vi "RTS Build Filename List.vi"(8 "Error In":errorcluster, 11 "RTS Config Setup":T1) -> (0 "Error Out":errorcluster, 3 "Full Filename List":string)   [LabVIEW 2016]
uses:
  Type Definitions/RTS Configuration Setup.ctl
  Type Definitions/RTS Wago Config.ctl
  Type Definitions/RTS APLUS Config.ctl
  Type Definitions/RTS Yokogawa MX Config.ctl
  Type Definitions/RTS Replay Server Control.ctl
  Type Definitions/RTS Server Configuration.ctl
  Type Definitions/RTS Station Settions TCP Comms.ctl
  Type Definitions/RTS Chamber Save Status.ctl
  Type Definitions/RTS Test Pattern.ctl
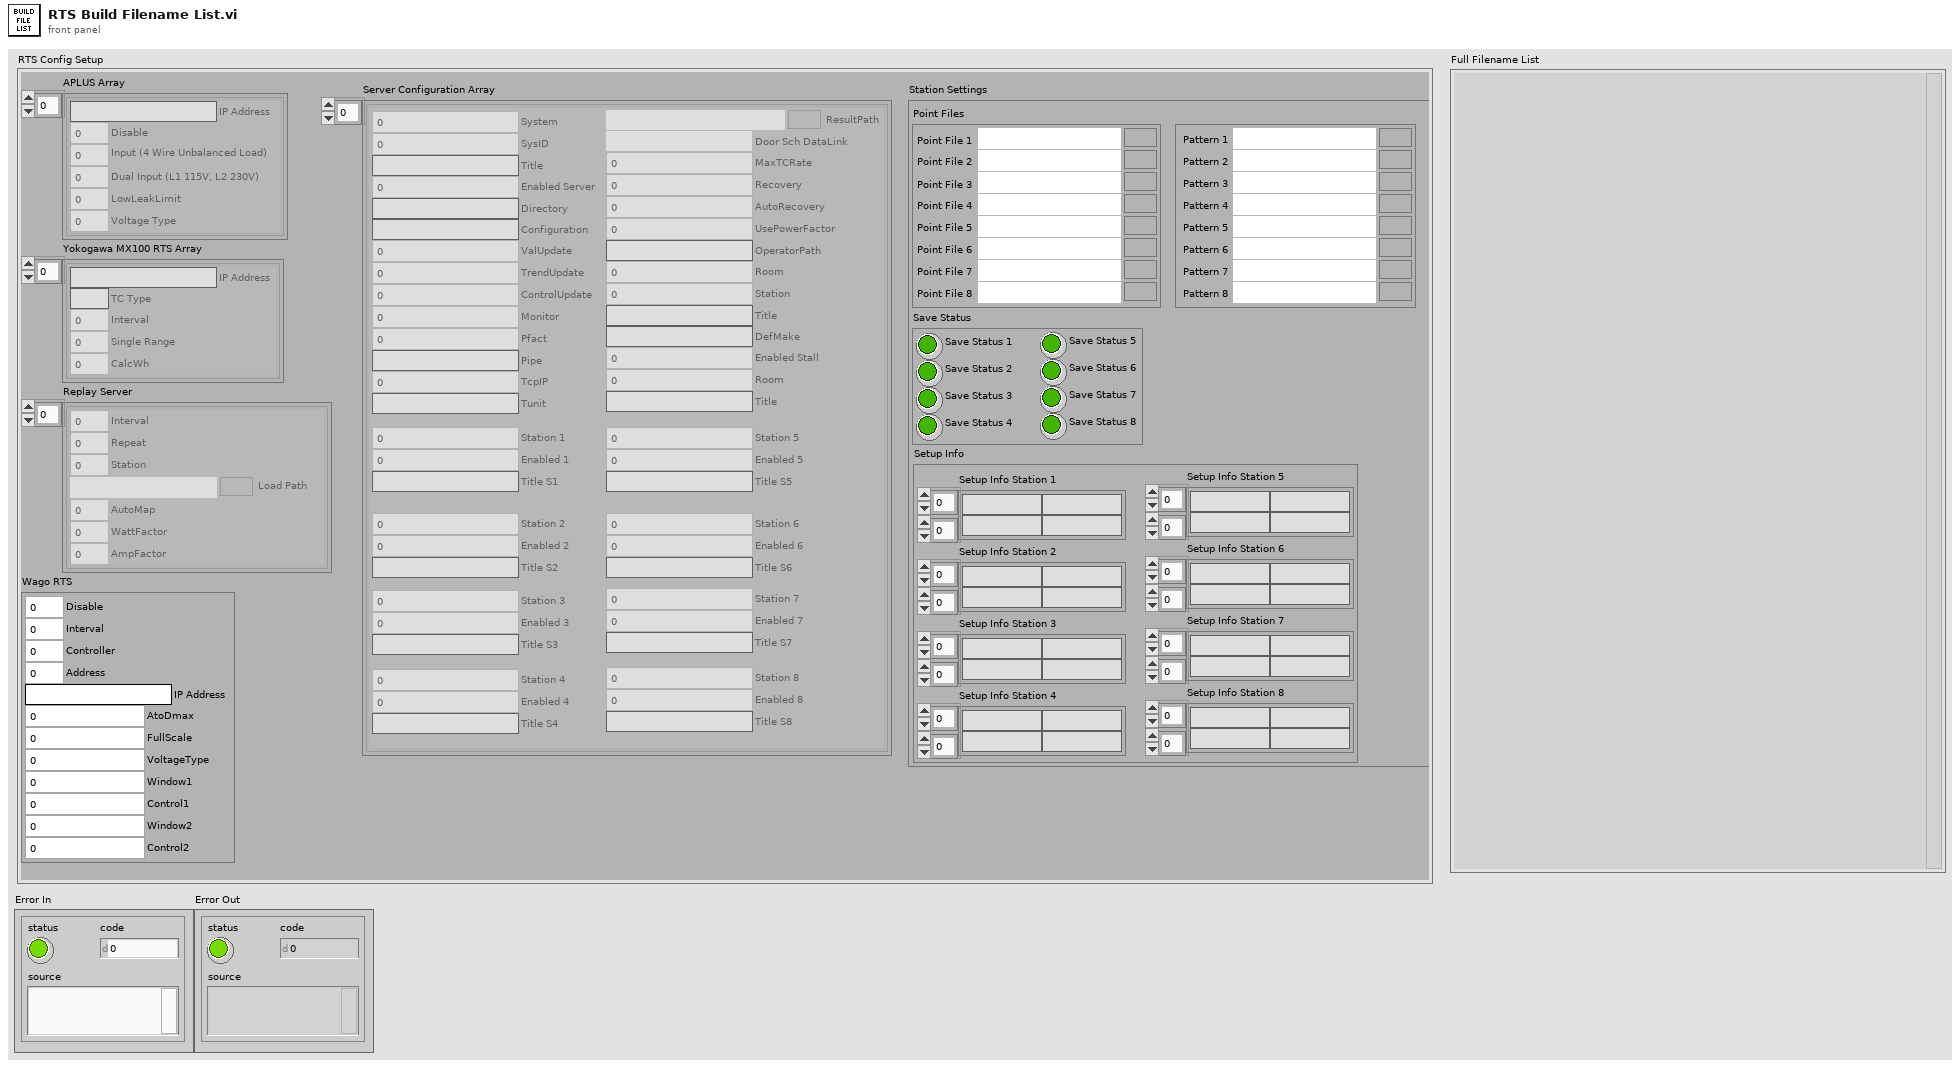
[diagram p1: front panel]
types:
  T1 = typedef "RTS Configuration Setup.ctl" = cluster{"Wago RTS":T2, "APLUS Array":T3[], "Yokogawa MX100 RTS Array":T4[], "Replay Server":T5[], "Server Configuration Array":T6[], "Station Settings":T7}
  T2 = typedef "RTS Wago Config.ctl" = cluster{"Disable":u16, "Interval":u16, "Controller":u16, "Address":u16, "IP Address":string, "AtoDmax":u16, "FullScale":u16, "VoltageType":u16, "Window1":u16, "Control1":u16, "Window2":u16, "Control2":u16}
  T3 = typedef "RTS APLUS Config.ctl" = cluster{"Disable":u16, "IP Address":string, "Input (4 Wire Unbalanced Load)":u16, "Dual Input (L1 115V, L2 230V)":u16, "LowLeakLimit":dbl, "Voltage Type":u16}
  T4 = typedef "RTS Yokogawa MX Config.ctl" = cluster{"IP Address":string, "TC Type":string, "Interval":u16, "Single Range":u16, "CalcWh":u16}
  T5 = typedef "RTS Replay Server Control.ctl" = cluster{"Interval":i16, "Repeat":u16, "Station":u16, "Load Path":path, "AutoMap":u16, "WattFactor":dbl, "AmpFactor":dbl}
  T6 = typedef "RTS Server Configuration.ctl" = cluster{"System":u16, "SysID":u16, "Title":string, "Enabled Server":u16, "Directory":string, "Configuration":string, "ValUpdate":u16, "TrendUpdate":u16, "ControlUpdate":u16, "Monitor":u16, "Pfact":u16, "Pipe":string, "TcpIP":u16, "Tunit":string, "ResultPath":path, "Door Sch DataLink":path, "MaxTCRate":u16, "Recovery":u16, "AutoRecovery":u16, "UsePowerFactor":u16, "OperatorPath":string, "Room":u16, "Station":u16, "Title":string, "DefMake":string, "Enabled Stall":u16, "Room":u16, "Title":string, "Station 1":u16, "Enabled 1":u16, "Station 2":u16, "Enabled 2":u16, "Station 3":u16, "Enabled 3":u16, "Station 4":u16, "Enabled 4":u16, "Station 5":u16, "Enabled 5":u16, "Station 6":u16, "Enabled 6":u16, "Station 7":u16, "Enabled 7":u16, "Station 8":u16, "Enabled 8":u16, "Title S1":string, "Title S2":string, "Title S3":string, "Title S5":string, "Title S6":string, "Title S7":string, "Title S8":string, "Title S4":string}
  T7 = typedef "RTS Station Settions TCP Comms.ctl" = cluster{"Point Files":cluster{"Point File 1":path, "Point File 2":path, "Point File 3":path, "Point File 4":path, "Point File 5":path, "Point File 6":path, "Point File 7":path, "Point File 8":path}, "Save Status":T8, "Setup Info":cluster{"Setup Info Station 1":string[][], "Setup Info Station 2":string[][], "Setup Info Station 3":string[][], "Setup Info Station 4":string[][], "Setup Info Station 5":string[][], "Setup Info Station 6":string[][], "Setup Info Station 7":string[][], "Setup Info Station 8":string[][]}, "Chamber Test Pattern":T9}
  T8 = typedef "RTS Chamber Save Status.ctl" = cluster{"Save Status 1":bool, "Save Status 2":bool, "Save Status 3":bool, "Save Status 4":bool, "Save Status 5":bool, "Save Status 6":bool, "Save Status 7":bool, "Save Status 8":bool}
  T9 = typedef "RTS Test Pattern.ctl" = cluster{" Pattern 1":path, "Pattern 2":path, "Pattern 3":path, "Pattern 4":path, "Pattern 5":path, "Pattern 6":path, "Pattern 7":path, "Pattern 8":path}
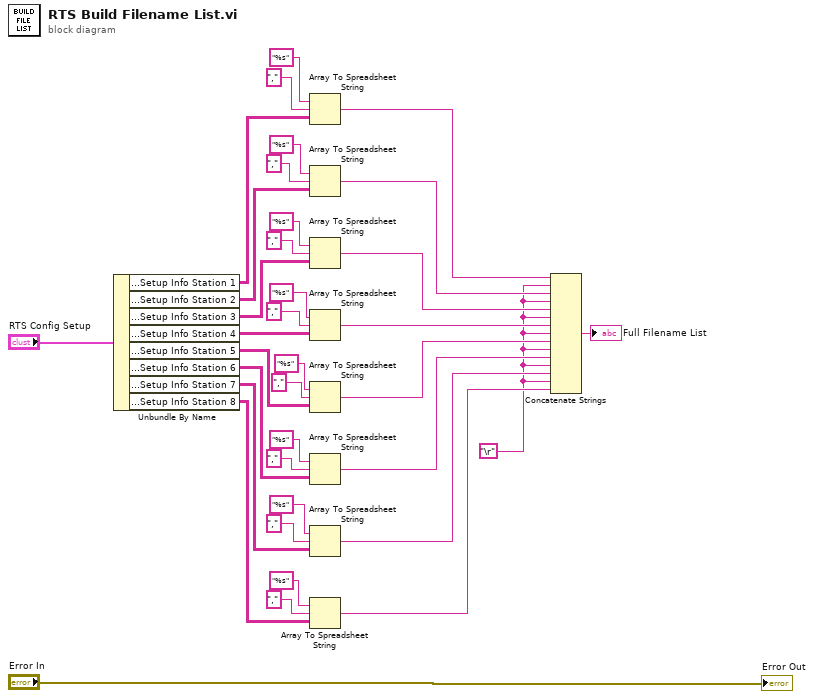
[diagram p0: block diagram]
diagram:
  w2 = "\r"
  n1 = Unbundle By Name("RTS Config Setup") -> ("Station Settings.Setup Info.Setup Info Station 1"=w15:string[][], "Station Settings.Setup Info.Setup Info Station 2"=w30:string[][], "Station Settings.Setup Info.Setup Info Station 3"=w31:string[][], "Station Settings.Setup Info.Setup Info Station 4"=w32:string[][], "Station Settings.Setup Info.Setup Info Station 5"=w33:string[][], "Station Settings.Setup Info.Setup Info Station 6"=w34:string[][], "Station Settings.Setup Info.Setup Info Station 7"=w35:string[][], "Station Settings.Setup Info.Setup Info Station 8"=w11:string[][])
  n2 = Array To Spreadsheet String(delimiter (Tab)=",", array=w15, 3:"%s" ("format string")) -> (spreadsheet string=w10:string)
  n3 = Array To Spreadsheet String(delimiter (Tab)=",", array=w30, 3:"%s" ("format string")) -> (spreadsheet string=w9:string)
  n4 = Array To Spreadsheet String(delimiter (Tab)=",", array=w31, 3:"%s" ("format string")) -> (spreadsheet string=w8:string)
  n5 = Array To Spreadsheet String(delimiter (Tab)=",", array=w32, 3:"%s" ("format string")) -> (spreadsheet string=w7:string)
  n6 = Array To Spreadsheet String(delimiter (Tab)=",", array=w33, 3:"%s" ("format string")) -> (spreadsheet string=w6:string)
  n7 = Array To Spreadsheet String(delimiter (Tab)=",", array=w34, 3:"%s" ("format string")) -> (spreadsheet string=w5:string)
  n8 = Array To Spreadsheet String(delimiter (Tab)=",", array=w35, 3:"%s" ("format string")) -> (spreadsheet string=w4:string)
  n9 = Array To Spreadsheet String(delimiter (Tab)=",", array=w11, 3:"%s" ("format string")) -> (spreadsheet string=w3:string)
  n10 = Concatenate Strings(w10, w2, w9, w2, w8, w2, w7, w2, w6, w2, w5, w2, w4, w2, w3) -> (→"Full Filename List":string)
  "Error Out" <- "Error In"
